vi "incrementProfileStepCounter.vi"(8 "error in (no error)":errorcluster, 11 "TestMonitor in":refnum<class "TestMonitor.lvclass">) -> (0 "error out":errorcluster, 2 "activeProfileStep":u32, 3 "TestMonitor out":refnum<class "TestMonitor.lvclass">)   [LabVIEW 2013, in "TestMonitor.lvclass"]
uses:
  TestMonitor.lvclass
  TestMonitor.lvclass/TestMonitor.ctl
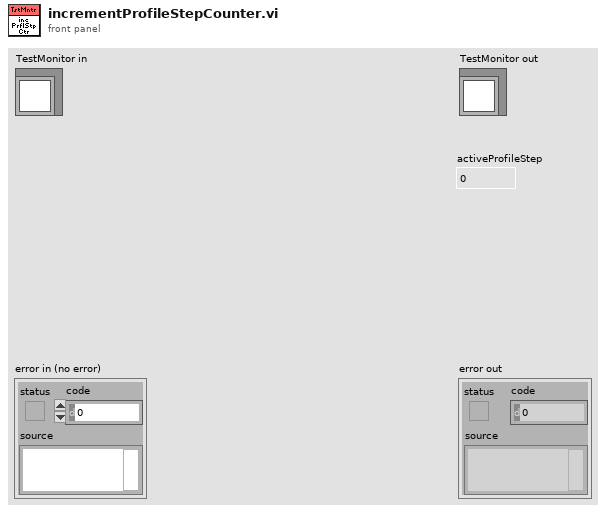
[diagram p1: front panel]
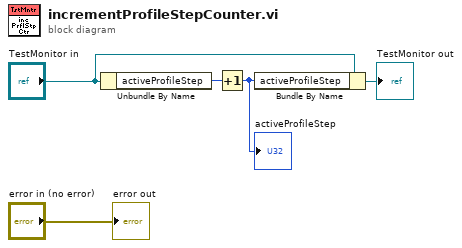
[diagram p0: block diagram]
diagram:
  n1 = Unbundle By Name("TestMonitor in") -> ("activeProfileStep"=w4:u32)
  n2 = Increment(x=w4) -> (x+1=w3:u32)
  "activeProfileStep" <- w3
  n3 = Bundle By Name(cluster="TestMonitor in", "activeProfileStep"=w3) -> (→"TestMonitor out":refnum<class "TestMonitor.lvclass">)
  "error out" <- "error in (no error)"
